vi "Get Brightenss Parameter.vi"(8 "error in (no error)":errorcluster, 11 "CameraStream in":refnum<class "CameraStream.lvclass">) -> (0 "error out":errorcluster, 2 "Value":i32, 3 "CameraStream (Duplicate)":refnum<class "CameraStream.lvclass">)   [LabVIEW 2020, in "g_ar_toolkit.capture.lvlib" / "CameraStream.lvclass"]
uses:
  CameraStream.lvclass
  Camera Parameters.ctl
  CameraStream.lvclass/CameraStream.ctl
  g_ar_toolkit.common/Module Path.vi
  <vilib>/Utility/error.llb/Error Cluster From Error Code.vi
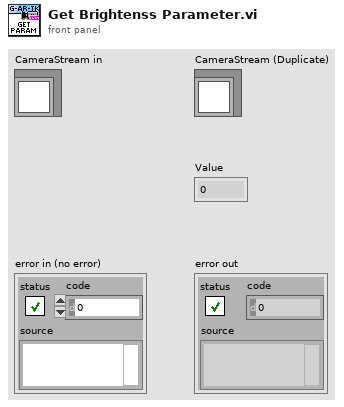
[diagram p1: front panel]
types:
  T1 = typedef "g_ar_toolkit.capture.lvlib/CameraStream.lvclass/Camera Parameters.ctl" = enum8{"EXPOSURE", "FOCUS", "ZOOM", "GAIN", "WHITE_BALANCE_TEMPERATURE", "BRIGHTNESS", "CONTRAST", "SATURATION", "GAMMA", "HUE", "SHARPNESS", "BACKLIGHT_COMPENSATION", "POWER_LINE_FREQUENCY"}
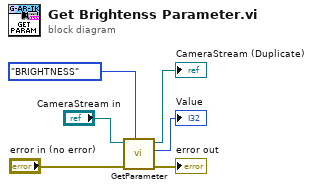
[diagram p0: block diagram]
diagram:
  n1 = call "GetParameter.vi"("Camera Parameter"=Camera_Parameters."BRIGHTNESS", "error in (no error)"="error in (no error)", "CameraStream in"="CameraStream in") -> ("error out"=→"error out":errorcluster, "Value"=→"Value":i32, "CameraStream (Duplicate)"=→"CameraStream (Duplicate)":refnum<class "CameraStream.lvclass">)  [unwired: 6 in]
